vi "Actor Core.vi"(8 "error in":errorcluster, 11 "Temperature Controller in":refnum<class "Temperature Controller.lvclass">) -> (0 "error out":errorcluster, 3 "Actor out":refnum<class "Actor.lvclass">)   [LabVIEW 2020, in "Temperature Controller.lvclass"]
doc: "(<B>Filename</B>: Actor Framework.lvlib:Actor.lvclass:Actor Core.vi)\n\nReceives messages to the actor, reacts to them, and initiates any error handling that may shut the actor down.\n\nDescendant classes may override this VI to append parallel tasks for the actor to complete while it handles messages. Overrides use the Call Parent Method node."
uses:
  Temperature Controller.lvclass
  opt/github/LabActor/Template Module/Template Module.lvclass
  Applications/National Instruments/LabVIEW 2020 64-bit/vi.lib/ActorFramework/Actor/Actor.lvclass
  <vilib>/ActorFramework/Actor/Actor.lvclass
  NHMFL_Core/Libraries/Instruments/Temperature Controller Driver/T controller configuration.ctl
  Template Module/Template Module.lvclass/Template Module.ctl
  <vilib>/ActorFramework/Actor/Actor.lvclass/Actor.ctl
  <vilib>/ActorFramework/Message Enqueuer/Message Enqueuer.lvclass/Message Enqueuer.ctl
  Instrument Actor Messages/Send Message Msg/Send Message Msg.lvclass/Send Message Msg.ctl
  Temperature Controller Messages/Set Point Msg/Set Point Msg.lvclass/Set Point Msg.ctl
  Template Module/Read stop event.vi
  <vilib>/ActorFramework/Message Enqueuer/Init from Existing Queue.vi
  <vilib>/ActorFramework/Message Enqueuer/Enqueue.vi
  Instrument Actor Messages/Send Message Msg/Send Message Msg.lvclass
  Applications/National Instruments/LabVIEW 2020 64-bit/vi.lib/ActorFramework/Message/Message.lvclass
  Temperature Controller Messages/Set Point Msg/Set Point Msg.lvclass
  <vilib>/ActorFramework/Message Priority Queue/Priority Enqueue.vi
  Instrument Actor/Instrument Actor.lvclass
  <vilib>/ActorFramework/Message Enqueuer/Message Enqueuer.lvclass
panel:
  in  "Send Command Button":bool
  in  "Command":string
  out "Name":string
  in  "Configuration":T1={"Record Channels"=["A"], "Add raw signal"=FALSE, "New set point"=0.0, "Record heater"=FALSE}
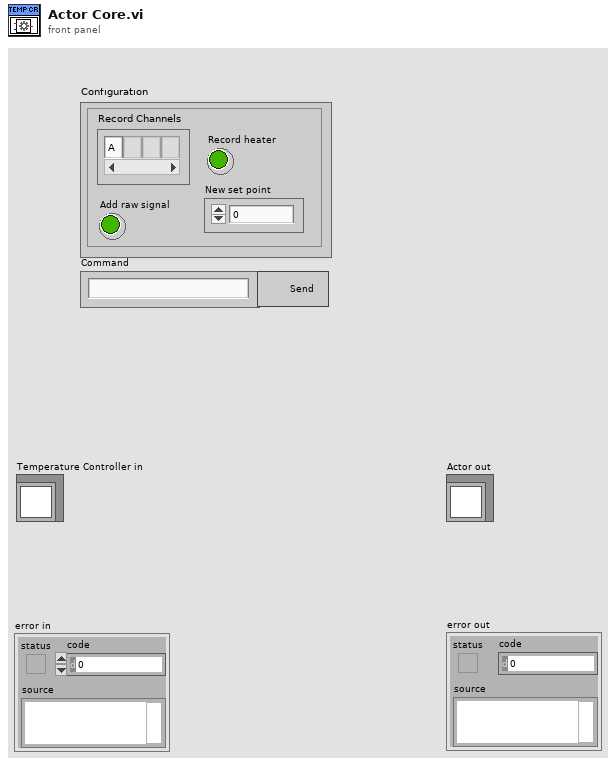
[diagram p1: front panel]
types:
  T1 = typedef "T controller configuration.ctl" = cluster{"Record Channels":string[], "Add raw signal":bool, "New set point":dbl, "Record heater":bool}
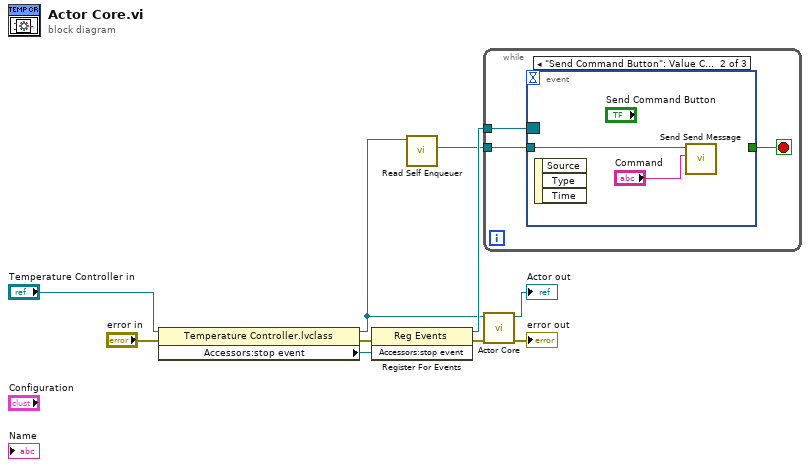
[diagram p0: block diagram]
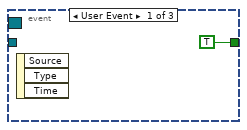
[diagram p2: hidden frame]
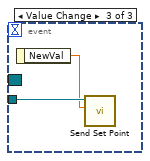
[diagram p3: hidden frame]
diagram:
  n1 = property class="Temperature Controller.lvclass"(reference="Temperature Controller in", error in="error in") -> (reference out=w2:refnum<class "Temperature Controller.lvclass">, error out=w4:errorcluster, "Accessors:stop event"=w6:refnum<user-event>)
  n2 = register-events(error in=w4, w6) -> (reference out=w5:refnum<event-registration>, error out=w3:errorcluster)  [unwired: 1 in]
  n3 = call <vilib>:"Read Self Enqueuer.vi"("Actor"=w2) -> ("Self Enqueuer"=w1:refnum<class "Message Enqueuer.lvclass">)  [unwired: 10 in]
  n4 = while {
    tunnel: w5 -> [w13]
    tunnel: w1 -> [w11]
    stop <- w12 stop-if-true
    n5 = event shown="[1] \"Send Command Button\": Value Change" {
      selector: w13 -> [_ _ _]
      dyn-events: _ -> [_ _ _]
      timeout: _ -> [_ _ _]
      tunnel: [TRUE _ _] -> w12
      tunnel: w11 -> [_ w16 w18]
      event User Event {
        n6 = event-data() -> ()  [unwired: 1 in, 3 out]
      }
      event "Send Command Button": Value Change {
        n7 = event-data() -> ()  [unwired: 1 in, 3 out]
        n8 = call "Send Send Message.vi"("Message"="Command", "Message Enqueuer"=w16) -> ()  [unwired: 8 in, 2 out]
      }
      event Value Change {
        n9 = event-data() -> ("NewVal"=w17:dbl)  [unwired: 1 in]
        n10 = call "Send Set Point.vi"("Set point"=w17, "Message Enqueuer"=w18) -> ()  [unwired: 8 in, 2 out]
      }
    }
  }
  n11 = call-parent "Actor Core.vi"("error in"=w3, "Measure Object in"=w2) -> ("error out"=→"error out":errorcluster, "Actor out"=→"Actor out":refnum<class "Actor.lvclass">)  [unwired: 8 in]
